vi "HP 53132A Config Channels.vi"(0 "VISA session":refnum<visa-resource-name>, 2 "channel":bool, 3 "Sensitivity":u16(ring)=2 items=["Sensitivity: low", "Sensitivity: med", "Sensitivity: hi"], 5 "error in (no error)":errorcluster, 10 "trigger":T1={FALSE, "PCT/trigger level"=50.0, "slope"=FALSE} {"PCT/trigger level" format="%.2f"}, 11 "100KHz Filter":bool, 14 "impedance":bool, 16 "coupling":bool, 17 "attenuation":bool) -> (15 "dup VISA session":refnum<visa-resource-name>, 19 "error out":errorcluster)   [LabVIEW 2012]
doc: "This VI configures a channel, such as trigger, sensitivity, imdedance, coupling, attenuation,, and filter.\n\nThe configuation for channel 3 is fixed:\n impedance: 50 ohms\n coupling: AC."
panel:
  # "2\n1"
  # "x10\nx1"
  # "50 ohms\n1M ohms"
  # "DC\nAC"
  # "Auto trigger:off + trigger level\nAuto trigger:on  + PCL level"
  # "neg (-)\npos (+)"
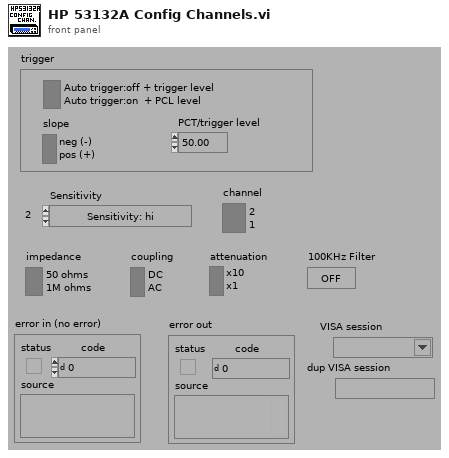
[diagram p1: front panel]
types:
  T1 = cluster{bool, "PCT/trigger level":dbl, "slope":bool}
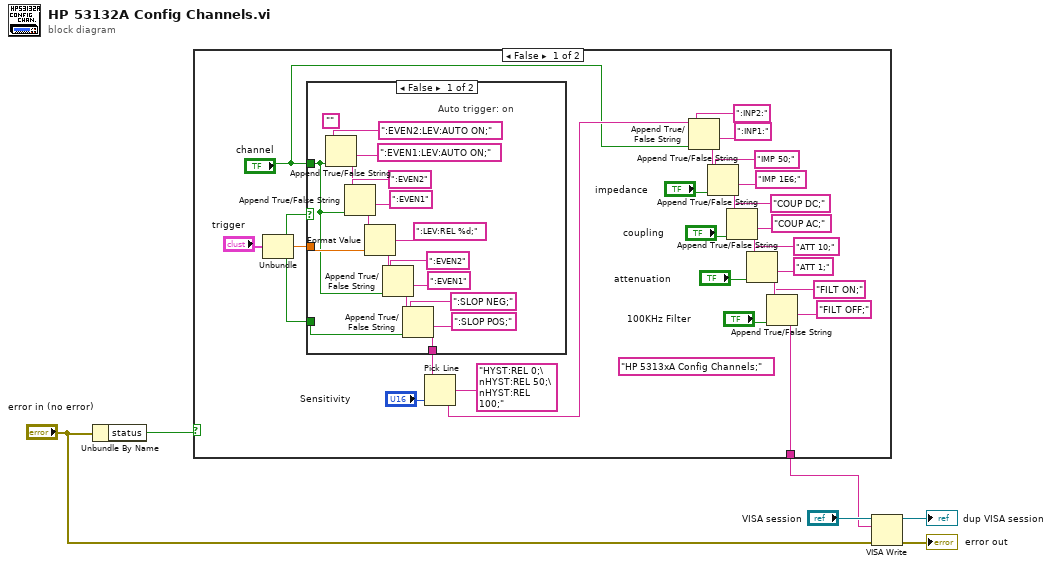
[diagram p0: block diagram]
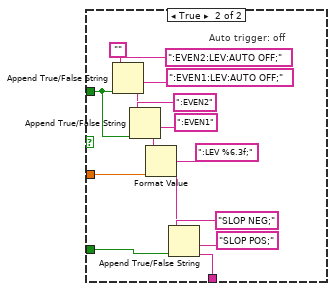
[diagram p2: hidden frame]
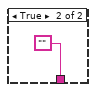
[diagram p3: hidden frame]
diagram:
  n1 = Unbundle By Name("error in (no error)") -> ("status"=w6:bool)
  n2 = case shown="False" w6 {
    tunnel: [w7 ""] -> w1
    frame False {
      (unwired) "HP 5313xA Config Channels;"
      n3 = Unbundle("trigger") -> (w24:bool, "PCT/trigger level"=w25:dbl, "slope"=w33:bool)
      n4 = case shown="False" w24 {
        tunnel: "channel" -> [w38 w59]
        tunnel: w25 -> [w43 w58]
        tunnel: [w35 w54] -> w34
        tunnel: w33 -> [w36 w53]
        frame False {
          # "Auto trigger: on"
          n5 = Append True/False String(1:w38, 2:":EVEN1:LEV:AUTO ON;", 3:":EVEN2:LEV:AUTO ON;", 4:"") -> (0:w47:string)
          n6 = Append True/False String(1:w38, 2:":EVEN1", 3:":EVEN2", 4:w47) -> (0:w42:string)
          n7 = Format Value(string ("")=w42, format string=":LEV:REL %d;", value (0)=w43) -> (output string=w39:string)
          n8 = Append True/False String(1:w38, 2:":EVEN1", 3:":EVEN2", 4:w39) -> (0:w37:string)
          n9 = Append True/False String(1:w36, 2:":SLOP POS;", 3:":SLOP NEG;", 4:w37) -> (0:w35:string)
        }
        frame True {
          # "Auto trigger: off"
          n10 = Append True/False String(1:w59, 2:":EVEN1:LEV:AUTO OFF;", 3:":EVEN2:LEV:AUTO OFF;", 4:"") -> (0:w61:string)
          n11 = Append True/False String(1:w59, 2:":EVEN1", 3:":EVEN2", 4:w61) -> (0:w64:string)
          n12 = Format Value(string ("")=w64, format string=":LEV %6.3f;", value (0)=w58) -> (output string=w55:string)
          n13 = Append True/False String(1:w53, 2:"SLOP POS;", 3:"SLOP NEG;", 4:w55) -> (0:w54:string)
        }
      }
      n14 = Pick Line(string ("")=w34, multi-line string="HYST:REL 0;\nHYST:REL 50;\nHYST:REL 100;", line index="Sensitivity") -> (output string=w32:string)
      n15 = Append True/False String(1:"channel", 2:":INP1:", 3:":INP2:", 4:w32) -> (0:w29:string)
      n16 = Append True/False String(1:"impedance", 2:"IMP 1E6;", 3:"IMP 50;", 4:w29) -> (0:w14:string)
      n17 = Append True/False String(1:"coupling", 2:"COUP AC;", 3:"COUP DC;", 4:w14) -> (0:w18:string)
      n18 = Append True/False String(1:"attenuation", 2:"ATT 1;", 3:"ATT 10;", 4:w18) -> (0:w22:string)
      n19 = Append True/False String(1:"100KHz Filter", 2:"FILT OFF;", 3:"FILT ON;", 4:w22) -> (0:w7:string)
    }
    frame True {
    }
  }
  n20 = VISA Write(VISA resource name="VISA session", write buffer=w1, error in (no error)="error in (no error)") -> (VISA resource name out=→"dup VISA session":refnum<visa-resource-name>, error out=→"error out":errorcluster)  [unwired: 1 out]
